vi "Move relative.vi"(8 "error in (no error)":errorcluster, 10 "Move array":dbl[](array[numeric]), 11 "ConfocalStage in":refnum<class "ConfocalStage.lvclass">) -> (0 "error out":errorcluster, 3 "ConfocalStage out":refnum<class "ConfocalStage.lvclass">)   [LabVIEW 2012, in "ConfocalStage.lvclass"]
uses:
  ConfocalStage.lvclass
  ConfocalStage.lvclass/ConfocalStage.ctl
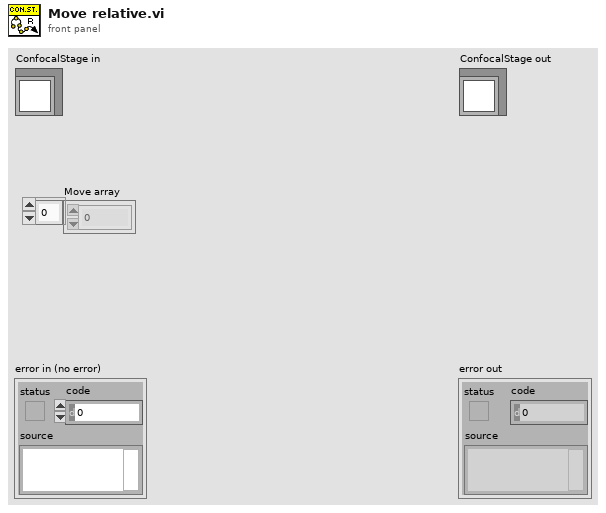
[diagram p1: front panel]
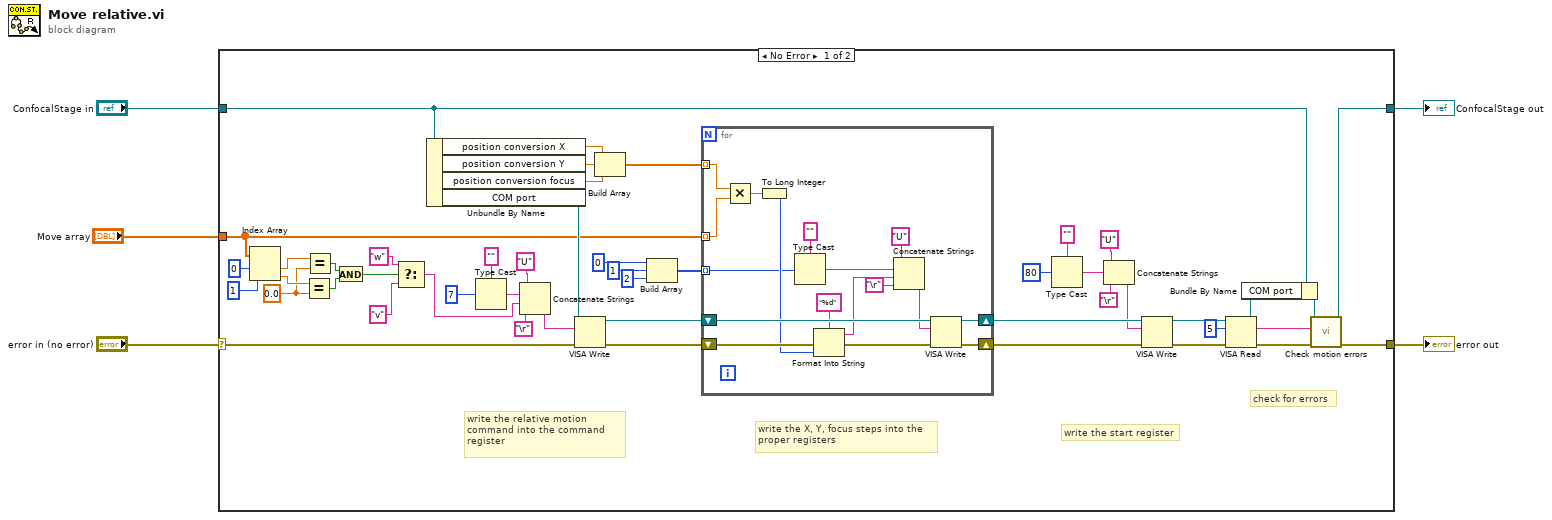
[diagram p0: block diagram]
diagram:
  n1 = case shown="No Error" "error in (no error)" {
    selector: "error in (no error)" -> [w44 w72]
    tunnel: [w25 w72] -> w4
    tunnel: [w23 w71] -> w2
    tunnel: "ConfocalStage in" -> [w24 w71]
    tunnel: "Move array" -> [w17 _]
    frame No Error {
      w12 = 0.0 ("y")
      # "check for errors"
      # "write the start register"
      # "write the X, Y, focus steps into the\nproper registers"
      # "write the relative motion\ncommand into the command\nregister"
      n2 = Index Array(array=w17, index #1=0 ("index"), index #2=1 ("index")) -> (element #1=w14:dbl, element #2=w13:dbl)
      n3 = Equal?(x=w13, y=w12) -> (x = y?=w10:bool)
      n4 = Equal?(x=w14, y=w12) -> (x = y?=w11:bool)
      n5 = And(x=w11, y=w10) -> (x .and. y?=w6:bool)
      n6 = Select(t="w", s=w6, f="v") -> (s? t:f=w8:string)
      n7 = Unbundle By Name(w24) -> ("position conversion X"=w53:dbl, "position conversion Y"=w52:dbl, "position conversion focus"=w51:dbl, "COM port"=w43:refnum<visa-resource-name>)
      n8 = Type Cast(type="", x=u8 7) -> (*(type *) &x=w48:string)
      n9 = Concatenate Strings("U", w48, w8, "\r") -> (w42:string)
      n10 = VISA Write(VISA resource name=w43, write buffer=w42, error in (no error)=w44) -> (VISA resource name out=w40:refnum<visa-resource-name>, error out=w41:errorcluster)  [unwired: 1 out]
      n11 = Build Array(w53, w52, w51) -> (w50:dbl[])
      n12 = Build Array(u8 0, u8 1, u8 2) -> (w36:u8[])
      n13 = for {
        tunnel: w17 -> [w70] mode=indexing
        tunnel: w50 -> [w69] mode=indexing
        shift-right: [w67] -> w34
        shift-left: w41 -> [w62]
        shift-right: [w55] -> w35
        shift-left: w40 -> [w66]
        tunnel: w36 -> [w57] mode=indexing
        n14 = Multiply(x=w69, y=w70) -> (x*y=w68:dbl)
        n15 = To Long Integer(number=w68) -> (32bit integer=w60:i32)
        n16 = Type Cast(type="", x=w57) -> (*(type *) &x=w64:string)
        n17 = Format Into String(format string="%d", error in=w62, w60) -> (resulting string=w58:string, error out=w61:errorcluster)  [unwired: 1 in]
        n18 = Concatenate Strings("U", w64, w58, "\r") -> (w56:string)
        n19 = VISA Write(VISA resource name=w66, write buffer=w56, error in (no error)=w61) -> (VISA resource name out=w55:refnum<visa-resource-name>, error out=w67:errorcluster)  [unwired: 1 out]
      }
      n20 = Type Cast(type="", x=u8 80) -> (*(type *) &x=w32:string)
      n21 = Concatenate Strings("U", w32, "\r") -> (w29:string)
      n22 = VISA Write(VISA resource name=w35, write buffer=w29, error in (no error)=w34) -> (VISA resource name out=w28:refnum<visa-resource-name>, error out=w45:errorcluster)  [unwired: 1 out]
      n23 = VISA Read(VISA resource name=w28, byte count=u32 5, error in (no error)=w45) -> (VISA resource name out=w21:refnum<visa-resource-name>, read buffer=w27:string, error out=w26:errorcluster)  [unwired: 1 out]
      n24 = Bundle By Name(cluster=w24, "COM port"=w21) -> (w22:refnum<class "ConfocalStage.lvclass">)
      n25 = call-dynamic "Check motion errors.vi"("error in (no error)"=w26, "VISA output string"=w27, "ConfocalStage in"=w22) -> ("error out"=w25:errorcluster, "ConfocalStage out"=w23:refnum<class "ConfocalStage.lvclass">)  [unwired: 7 in]
    }
    frame Error {
    }
  }
  "error out" <- w4
  "ConfocalStage out" <- w2
